vi "initializeAccelerometers.vi"(8 "ErrorIn":errorcluster, 11 "I2C Ref In":T1={"myRIO Reference"={"myRIO Model"=enum."Unknown", "myRIO Hardware Reference"={"Generic FPGA Reference"=refnum, "Allow multiple opens"=FALSE}}, "I2C Channels Enum"=enum."Not Connected", "I2C Configuration"={"I2C Transfer Rate"=enum."Fast mode (400 kbps)"}}) -> (0 "ErrorOut":errorcluster, 3 "I2C Ref Out":T1)   [LabVIEW 2019]
uses:
  <vilib>/myRIO/Instrument Drivers/Onboard IO/I2C/typedefs/I2C Reference.ctl
  <vilib>/myRIO/Common/Instrument Driver Framework/Utilities/typedefs/myRIO Generic Hardware Reference.ctl
  <vilib>/myRIO/Common/Instrument Driver Framework/Utilities/typedefs/Hardware Version Enum.ctl
  <vilib>/myRIO/Common/Instrument Driver Framework/Utilities/typedefs/myRIO v1.0 Reference.ctl
  <vilib>/myRIO/Common/Instrument Driver Framework/Utilities/typedefs/Generic FPGA Reference.ctl
  <vilib>/myRIO/Common/Instrument Driver Framework/myRIO v1.0/I2C/typedefs/I2C Channels Enum.ctl
  <vilib>/myRIO/Instrument Drivers/Onboard IO/I2C/typedefs/I2C Configuration.ctl
  <vilib>/myRIO/Instrument Drivers/Onboard IO/I2C/typedefs/I2C Transfer Rate.ctl
  <vilib>/Utility/error.llb/Error Cluster From Error Code.vi
  <vilib>/myRIO/Common/Instrument Driver Framework/myRIO v1.0/I2C/vis/myRIO v1.0 Write I2C.vi
  <vilib>/myRIO/Common/Instrument Driver Framework/myRIO v1.0/I2C/vis/myRIO v1.0 Read I2C.vi
  <vilib>/myRIO/Instrument Drivers/Onboard IO/I2C/I2C.lvlib
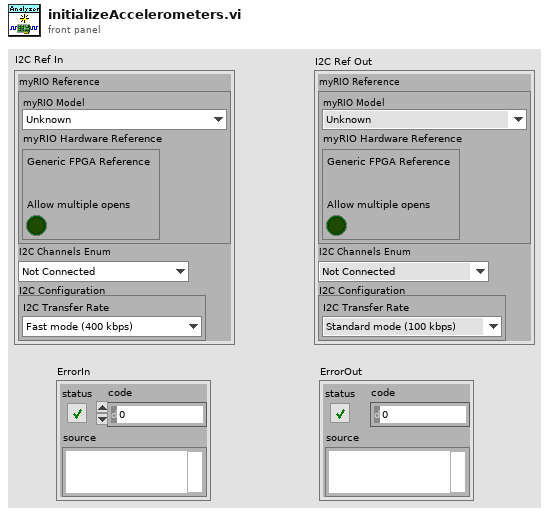
[diagram p1: front panel]
types:
  T1 = typedef "I2C.lvlib/I2C Reference.ctl" = cluster{"myRIO Reference":T2, "I2C Channels Enum":T6, "I2C Configuration":T7}
  T2 = typedef "myRIO Generic Hardware Reference.ctl" = cluster{"myRIO Model":T3, "myRIO Hardware Reference":T4}
  T3 = typedef "Hardware Version Enum.ctl" = enum16{"Unknown", "myRIO-1900", "myRIO-1950", "roboRIO", "NI ELVIS RIO CM", "ELVIS III"}
  T4 = typedef "myRIO v1.0 Reference.ctl" = cluster{"Generic FPGA Reference":T5, "Allow multiple opens":bool}
  T5 = typedef "Generic FPGA Reference.ctl" = refnum<k20>
  T6 = typedef "I2C Channels Enum.ctl" = enum16{"Not Connected", "A/I2C", "B/I2C", "I2C/I2C"}
  T7 = typedef "I2C.lvlib/I2C Configuration.ctl" = cluster{"I2C Transfer Rate":T8}
  T8 = typedef "I2C.lvlib/I2C Transfer Rate.ctl" = enum16{"Standard mode (100 kbps)", "Fast mode (400 kbps)"}
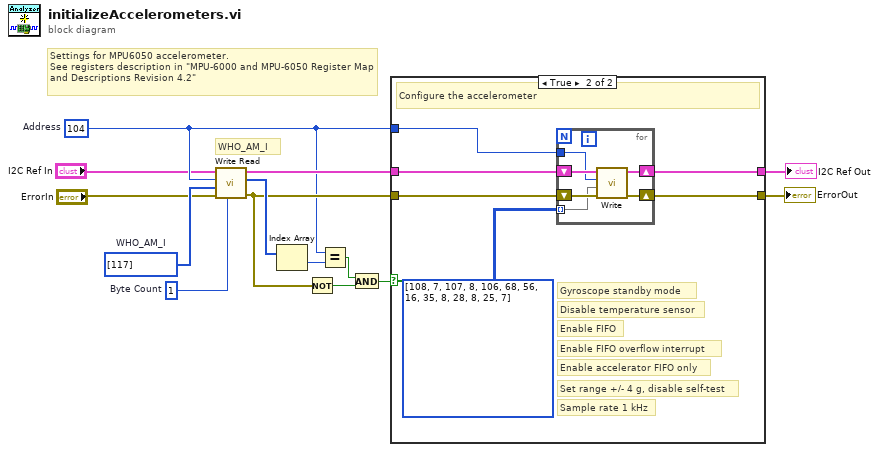
[diagram p0: block diagram]
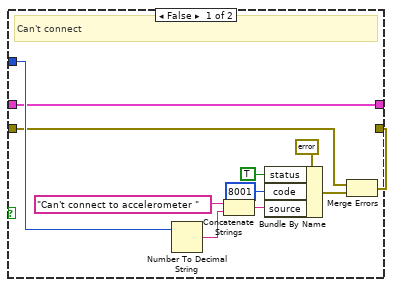
[diagram p2: hidden frame]
diagram:
  w6 = u8 104  # Address
  w12 = u32 1  # Byte Count
  w11 = u8[] [117]  # WHO_AM_I
  # "Settings for MPU6050 accelerometer.\nSee registers description in \"MPU-6000 and MPU-6050 Register Map and Descriptions Revision 4.2\""
  # "WHO_AM_I"
  n1 = call <vilib>:"Write Read.vi"("Byte Count"=w12, "error in (no error)"="ErrorIn", "Bytes to Write"=w11, "Slave Address (7-bit)"=w6, "I2C Ref In"="I2C Ref In") -> ("error out"=w8:errorcluster, "Bytes Read"=w13:u8[], "I2C Ref Out"=w10:T1)  [unwired: 3 in]
  n2 = Index Array(array=w13) -> (element=w14:u8)  [unwired: 1 in]
  n3 = Not(x=w8) -> (.not. x?=w7:bool)
  n4 = Equal?(x=w6, y=w14) -> (x = y?=w9:bool)
  n5 = And(x=w9, y=w7) -> (x .and. y?=w5:bool)
  n6 = case shown="True" w5 {
    tunnel: w6 -> [w23 w28]
    tunnel: w10 -> [w15 w31]
    tunnel: w8 -> [w18 w30]
    tunnel: [w16 w27] -> w4
    tunnel: [w15 w26] -> w3
    frame False {
      # "Can't connect"
      n7 = Number To Decimal String(number=w23) -> (decimal integer string=w20:string)  [unwired: 1 in]
      n8 = Concatenate Strings("Can't connect to accelerometer " ("source"), w20) -> (w22:string)
      n9 = Bundle By Name(cluster=errorcluster {"status"=FALSE, "code"=0, "source"=""} ("error constant"), "status"=TRUE, "code"=8001, "source"=w22) -> (w17:errorcluster)
      n10 = Merge Errors(w18, w17) -> (w16:errorcluster)
    }
    frame True {
      # "Sample rate 1 kHz"
      # "Enable accelerator FIFO only"
      # "Disable temperature sensor"
      # "Gyroscope standby mode"
      # "Set range +/- 4 g, disable self-test"
      # "Enable FIFO"
      # "Enable FIFO overflow interrupt"
      # "Configure the accelerometer"
      n11 = for {
        shift-right: [w34] -> w27
        shift-left: w30 -> [w37]
        shift-right: [w35] -> w26
        shift-left: w31 -> [w36]
        tunnel: u8[][] [[108, 7], [107, 8], [106, 68], [56, 16], [35, 8], [28, 8], [25, 7]] ("Bytes to Write") -> [w33] mode=indexing
        tunnel: w28 -> [w32]
        n12 = call <vilib>:"Write.vi"("error in (no error)"=w37, "Bytes to Write"=w33, "Slave Address (7-bit)"=w32, "I2C Ref In"=w36) -> ("error out"=w34:errorcluster, "I2C Ref Out"=w35:T1)  [unwired: 6 in]
      }
    }
  }
  "ErrorOut" <- w4
  "I2C Ref Out" <- w3
